vi "test Get-Set-Get HW Configuration File Paths.vi"(8 "error in":errorcluster, 11 "TestCase in":refnum<class "Scripting.lvclass">) -> (0 "error out":errorcluster, 3 "TestCase out":refnum<class "Scripting.lvclass">)   [LabVIEW 2020, in "Scripting.lvclass"]
uses:
  Scripting.lvclass
  <vilib>/addons/_JKI Toolkits/VI Tester/TestCase.llb/TestCase.lvclass
  Scripting/Ballard ARINC 429 Scripting.lvlib
  niveristand-custom-device-testing-tools/VeriStandTestUtilities/VeriStandTestUtilities.lvlib
  C:/Program Files (x86)/National Instruments/LabVIEW 2020/vi.lib/addons/_JKI Toolkits/VI Tester/TestCase.llb/TestCase.lvclass
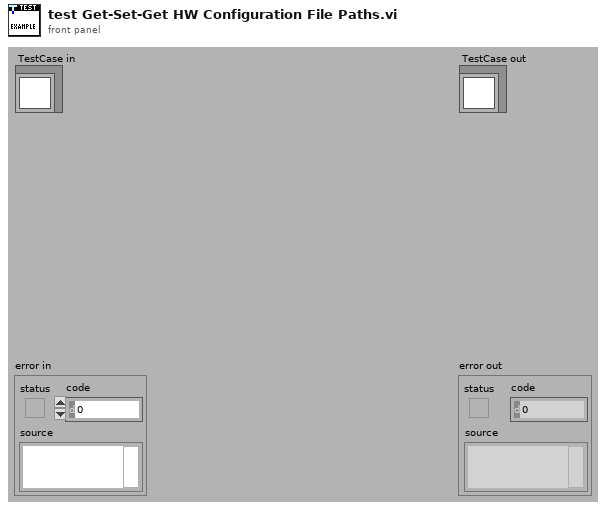
[diagram p1: front panel]
types:
  T1 = typedef "Custom Device API.lvlib/Custom Device Item Ref.ctl" = u64
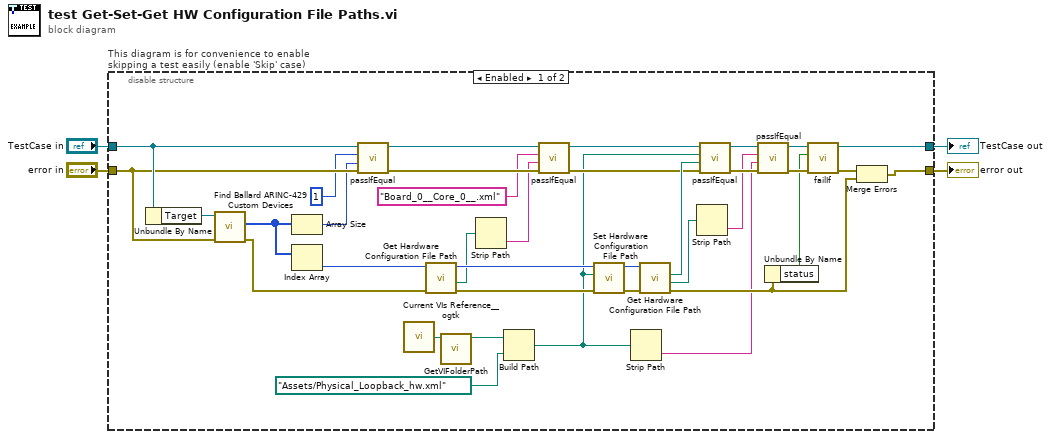
[diagram p0: block diagram]
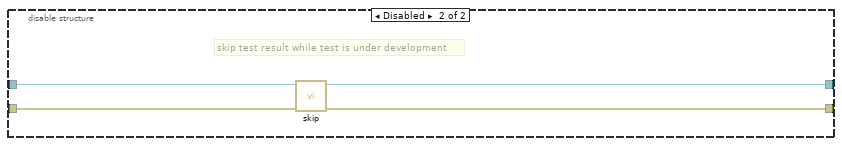
[diagram p2: hidden frame]
diagram:
  n1 = disable-structure "This diagram is for convenience to enable skipping a test easily (enable 'Skip' case)" shown="Enabled" {
    disable-tunnel: "TestCase in" -> [w39 w44]
    disable-tunnel: [w29 w42] -> w1
    disable-tunnel: [w35 w43] -> w3
    disable-tunnel: "error in" -> [w38 w41]
    frame Enabled {
      n2 = Unbundle By Name(w39) -> ("Target"=w40:refnum<k24>)
      n3 = call "Find Ballard ARINC-429 Custom Devices.vi"("error in"=w38, "target in"=w40) -> ("error out"=w7:errorcluster, "Ballard ARINC 429 custom devices"=w5:u64[])  [unwired: 7 in, 1 out]
      n4 = Array Size(array=w5) -> (size(s)=w36:i32)
      n5 = Index Array(array=w5) -> (element=w6:u64)  [unwired: 1 in]
      n6 = call-dynamic "passIfEqual.vi"("error in (no error)"=w38, "y"=w36, "x"=1 ("size(s)"), "TestCase in"=w39) -> ("error out"=w18:errorcluster, "TestCase out"=w17:refnum<class "Scripting.lvclass">)  [unwired: 6 in]
      n7 = call <userlib>:"Current VIs Reference__ogtk.vi"() -> ("Current VI's reference"=w10:refnum<vi>)  [unwired: 5 in]
      n8 = call "Get Hardware Configuration File Path.vi"("error in"=w7, "custom device ref"=w6) -> ("error out"=w25:errorcluster, "RTDestination"=w14:path, "custom device ref out"=w28:T1)  [unwired: 6 in, 1 out]
      n9 = call "GetVIFolderPath.vi"("VI Reference in"=w10) -> ("VI Folder Path out"=w11:path)  [unwired: 9 in, 1 out]
      n10 = Strip Path(path=w14) -> (name=w13:string)  [unwired: 1 out]
      n11 = Build Path(base path=w11, name or relative path=path "Assets/Physical_Loopback_hw.xml" ("Absolute or Relative Path")) -> (appended path=w8:path)
      n12 = call-dynamic "passIfEqual.vi"("error in (no error)"=w18, "y"=w13, "x"="Board_0__Core_0__.xml" ("name"), "TestCase in"=w17) -> ("error out"=w15:errorcluster, "TestCase out"=w16:refnum<class "Scripting.lvclass">)  [unwired: 6 in]
      n13 = call "Set Hardware Configuration File Path.vi"("error in"=w25, "path"=w8, "custom device ref"=w28) -> ("error out"=w26:errorcluster, "custom device ref out"=w27:T1)  [unwired: 7 in]
      n14 = Strip Path(path=w8) -> (name=w20:string)  [unwired: 1 out]
      n15 = call "Get Hardware Configuration File Path.vi"("error in"=w26, "custom device ref"=w27) -> ("error out"=w23:errorcluster, "RTDestination"=w22:path, "path"=w19:path)  [unwired: 6 in, 1 out]
      n16 = Strip Path(path=w22) -> (name=w21:string)  [unwired: 1 out]
      n17 = call-dynamic "passIfEqual.vi"("error in (no error)"=w15, "y"=w19, "x"=w8, "TestCase in"=w16) -> ("error out"=w33:errorcluster, "TestCase out"=w34:refnum<class "Scripting.lvclass">)  [unwired: 6 in]
      n18 = call-dynamic "passIfEqual.vi"("error in (no error)"=w33, "y"=w20, "x"=w21, "TestCase in"=w34) -> ("error out"=w31:errorcluster, "TestCase out"=w30:refnum<class "Scripting.lvclass">)  [unwired: 6 in]
      n19 = Unbundle By Name(w23) -> ("status"=w24:bool)
      n20 = call-dynamic "failIf.vi"("error in (no error)"=w31, "fail"=w24, "TestCase in"=w30) -> ("error out"=w32:errorcluster, "TestCase out"=w29:refnum<class "Scripting.lvclass">)  [unwired: 7 in]
      n21 = Merge Errors(w32, w23) -> (w35:errorcluster)
    }
    frame Disabled {
      # "skip test result while test is under development"
      n22 = call <vilib>:"skip.vi"("error in (no error)"=w41, "TestCase in"=w44) -> ("error out"=w43:errorcluster, "TestCase out"=w42:refnum<class "Scripting.lvclass">)  [unwired: 8 in]
    }
  }
  "error out" <- w3
  "TestCase out" <- w1
